vi "Create.vi"(9 "Channel Name":string, 10 "Channel Writer":u64, 11 "Nominal Streaming":refnum<class "Stream.lvclass">) -> (3 "Channel":refnum<class "Channel.lvclass">)   [LabVIEW 2020, in "Nominal Streaming.lvlib" / "Channel.lvclass"]
uses:
  Channel.lvclass
  Stream/Stream.lvclass
  Channel.lvclass/Channel.ctl
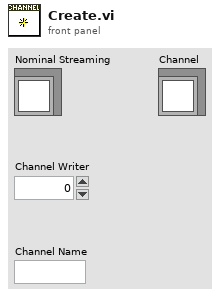
[diagram p1: front panel]
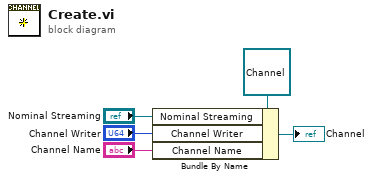
[diagram p0: block diagram]
diagram:
  n1 = Bundle By Name(cluster=refnum<class "Channel.lvclass"> refnum ("Channel"), "Nominal Streaming"="Nominal Streaming", "Channel Writer"="Channel Writer", "Channel Name"="Channel Name") -> (→"Channel":refnum<class "Channel.lvclass">)
